vi "Card Used array.vi"() -> ()   [LabVIEW 2014]
panel:
  out "Card used array":dbl[](array[numeric])
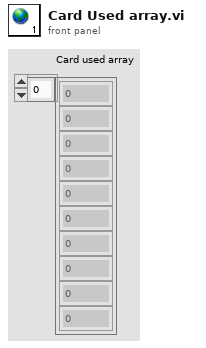
[diagram p1: front panel]
diagram:
